vi "CU_trainSVM.vi"(6 "Train Data":T1, 8 "error in (no error)":errorcluster, 9 "Indices":i8[](array[numeric]), 10 "Nu Value":dbl, 11 "ClassifierClass in":refnum<class "ClassifierClass.lvclass">) -> (0 "error out":errorcluster, 2 "Classifier Session out":T2, 3 "ClassifierClass out":refnum<class "ClassifierClass.lvclass">)   [LabVIEW 2016, in "Classifier.lvlib" / "ClassifierClass.lvclass"]
uses:
  ClassifierClass.lvclass
  <vilib>/vision/Classification.llb/IMAQ Classifier SVM Training Results.ctl
  <vilib>/vision/Classification.llb/IMAQ Classifier Session.ctl
  CU_DataTypes.ctl
  ClassifierClass.lvclass/ClassifierClass.ctl
  <vilib>/vision/NI_Vision_Development_Module.lvlib
  Classifier.lvlib
panel:
  out "Training Results":T3[](array[typedef]) {"Standard Deviation" format="%.2f"}
  # "This VI is a part of BCI Design library, http://www.ru-bci.org \nCopyright © 2020, Sotnikov Peter, All rights reserved. License: CC BY-NC 4.0"
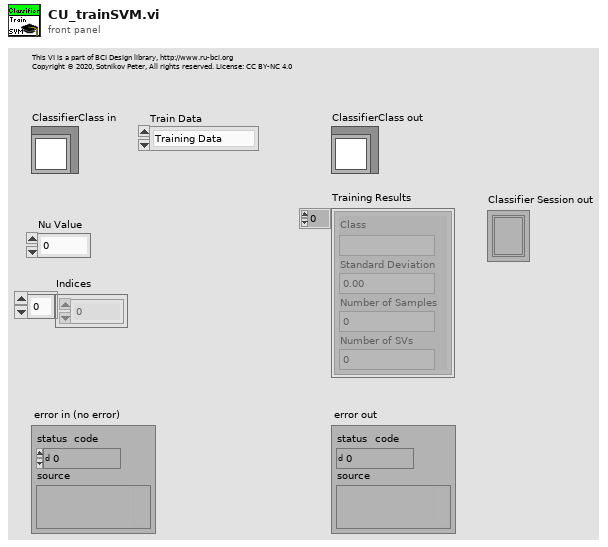
[diagram p1: front panel]
types:
  T1 = typedef "Classifier.lvlib/CU_DataTypes.ctl" = enum16{"Training Data", "Test Data", "Training Data (cross-check)", "Test Data (cross-check)"}
  T2 = typedef "IMAQ Classifier Session.ctl" = refnum<k1>
  T3 = typedef "IMAQ Classifier SVM Training Results.ctl" = cluster{"Class":string, "Standard Deviation":sgl, "Number of Samples":i32, "Number of SVs":i32}
  T4 = typedef "XML_EEG_Features.lvlib/XML_FF_Trial.ctl" = cluster{"ClassLabel":string, "FeatureVector":dbl[]}
  T5 = typedef "IMAQ SVM Kernel Options.ctl" = cluster{"Kernel":enum32{"Linear", "Polynomial", "Gaussian", "RBF"}, "Degree":i32, "Gamma":dbl, "Coefficient":dbl, "Sigma":dbl, "Cache(MB)":dbl}
  T6 = typedef "IMAQ SVM Model Options.ctl" = cluster{"SVM Model":enum32{"C-SVC", "nu-SVC", "One Class"}, "Tolerance":dbl, "Max. Iteration":i32, "Nu":dbl, "Shrinking":bool, "Cost":dbl, "Weighted Cost":cluster{"Label":string, "Weight":dbl}[]}
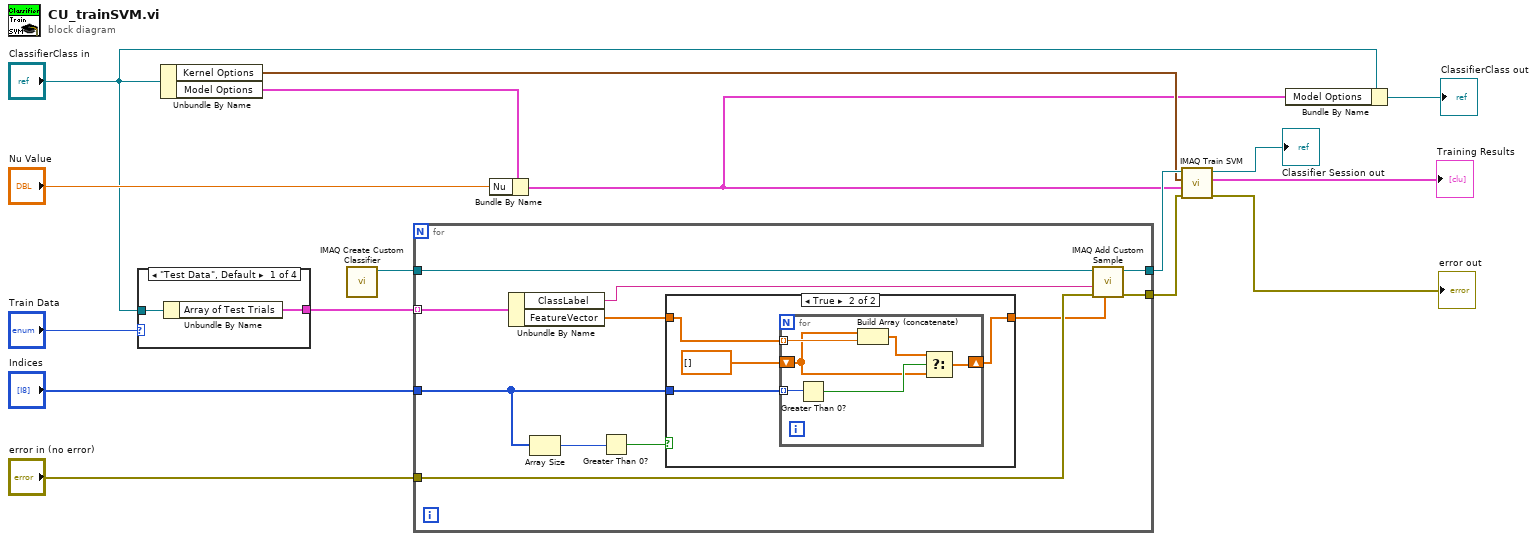
[diagram p0: block diagram]
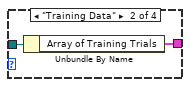
[diagram p2: hidden frame]
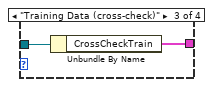
[diagram p3: hidden frame]
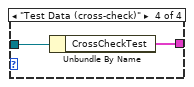
[diagram p4: hidden frame]
diagram:
  n1 = case shown="\"Test Data\", Default" "Train Data" {
    tunnel: "ClassifierClass in" -> [w18 w20 w22 w24]
    tunnel: [w17 w19 w21 w23] -> w1
    frame "Test Data", Default {
      n2 = Unbundle By Name(w18) -> ("Array of Test Trials"=w17:T4[])
    }
    frame "Training Data" {
      n3 = Unbundle By Name(w20) -> ("Array of Training Trials"=w19:T4[])
    }
    frame "Training Data (cross-check)" {
      n4 = Unbundle By Name(w22) -> ("CrossCheckTrain"=w21:T4[])
    }
    frame "Test Data (cross-check)" {
      n5 = Unbundle By Name(w24) -> ("CrossCheckTest"=w23:T4[])
    }
  }
  n6 = Unbundle By Name("ClassifierClass in") -> ("Kernel Options"=w7:T5, "Model Options"=w16:T6)
  n7 = call "IMAQ Create Custom Classifier"() -> ("Classifier Session"=w8:T2)  [unwired: 10 in, 1 out]
  n8 = for {
    tunnel: w1 -> [w35] mode=indexing
    tunnel: w8 -> [w34]
    tunnel: "error in (no error)" -> [w32]
    tunnel: "Indices" -> [w28]
    tunnel: [w27] -> w10
    tunnel: [w26] -> w9
    n9 = Unbundle By Name(w35) -> ("ClassLabel"=w33:string, "FeatureVector"=w29:dbl[])
    n10 = Array Size(array=w28) -> (size(s)=w31:i32)
    n11 = Greater Than 0?(x=w31) -> (x > 0?=w30:bool)
    n12 = case shown="True" w30 {
      tunnel: w29 -> [w36 w40]
      tunnel: [w36 w37] -> w25
      tunnel: w28 -> [_ w39]
      frame False {
      }
      frame True {
        n13 = for {
          tunnel: w40 -> [w43] mode=indexing
          tunnel: w39 -> [w46] mode=indexing
          shift-right: [w45] -> w37
          shift-left: dbl[] [] -> [w41]
          n14 = Greater Than 0?(x=w46) -> (x > 0?=w44:bool)
          n15 = Build Array (concatenate)(w41, w43) -> (w42:dbl[])
          n16 = Select(t=w42, s=w44, f=w41) -> (s? t:f=w45:dbl[])
        }
      }
    }
    n17 = call "IMAQ Add Custom Sample"("Feature Vector"=w25, "error in (no error)"=w32, "Class"=w33, "Classifier Session"=w34) -> ("error out"=w27:errorcluster, "Classifier Session (dup)"=w26:T2)  [unwired: 6 in]
  }
  n18 = Bundle By Name(cluster=w16, "Nu"="Nu Value") -> (w6:T6)
  n19 = call "IMAQ Train SVM"("error in (no error)"=w10, "Model Options"=w6, "Kernel Options"=w7, "Classifier Session"=w9) -> ("error out"=→"error out":errorcluster, "Training Results"=→"Training Results":T3[], "Classifier Session (dup)"=→"Classifier Session out":T2)  [unwired: 4 in, 1 out]
  n20 = Bundle By Name(cluster="ClassifierClass in", "Model Options"=w6) -> (→"ClassifierClass out":refnum<class "ClassifierClass.lvclass">)
